vi "Excel Secondary Header Prep.vi"(0 "RefCellsIn":refnum<k7>, 7 "[IndexPageStarts]":i32[](array[numeric]), 11 "ErrorIn":errorcluster) -> (4 "RefCellsOut":refnum<k7>, 15 "ErrorOut":errorcluster)   [LabVIEW 2013]
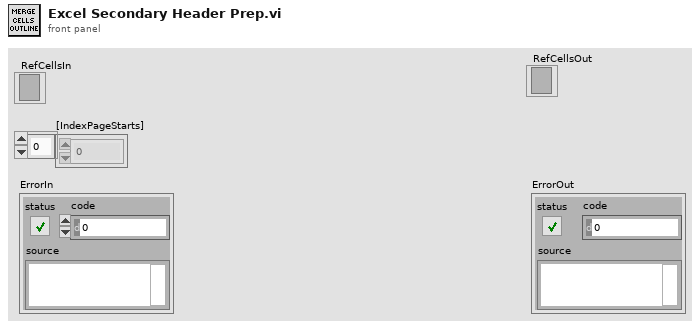
[diagram p1: front panel]
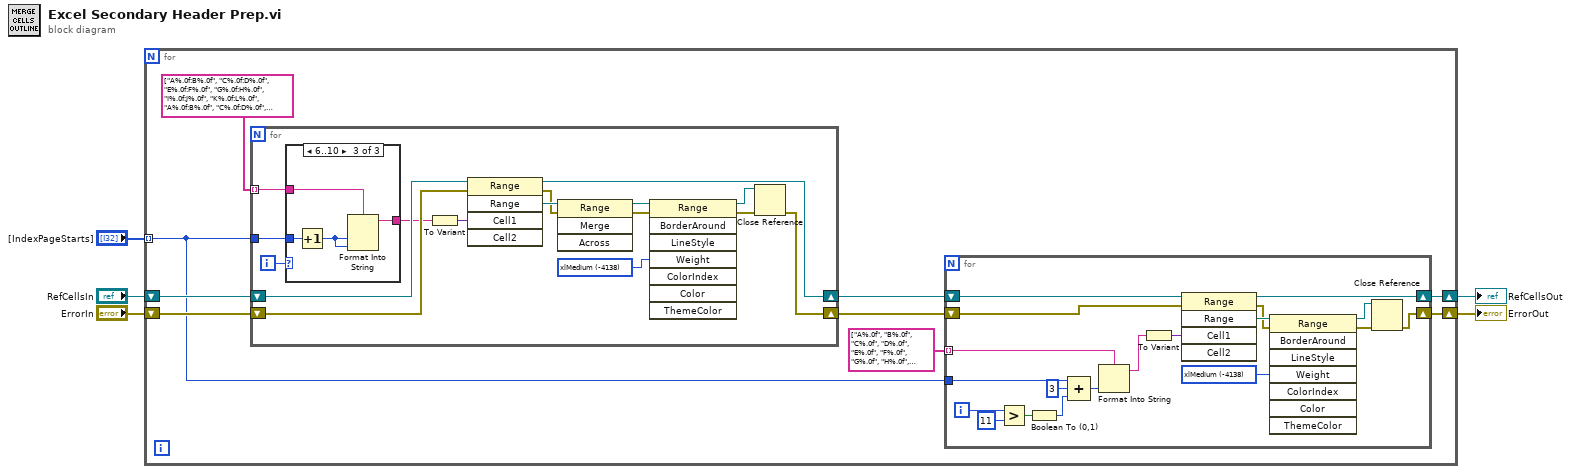
[diagram p0: block diagram]
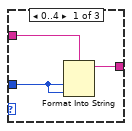
[diagram p2: hidden frame]
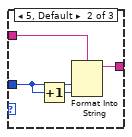
[diagram p3: hidden frame]
diagram:
  n1 = for {
    tunnel: "[IndexPageStarts]" -> [w12] mode=indexing
    shift-right: [w9] -> w3
    shift-left: "RefCellsIn" -> [w14]
    shift-right: [w8] -> w2
    shift-left: "ErrorIn" -> [w13]
    n2 = for {
      tunnel: string[] ["A%.0f:B%.0f", "C%.0f:D%.0f", "E%.0f:F%.0f", "G%.0f:H%.0f", "I%.0f:J%.0f", "K%.0f:L%.0f", "A%.0f:B%.0f", "C%.0f:D%.0f", "E%.0f:F%.0f", "G%.0f:H%.0f", "I%.0f:J%.0f"] -> [w48] mode=indexing
      tunnel: w12 -> [w47]
      shift-right: [w43] -> w11
      shift-left: w14 -> [w44]
      shift-right: [w42] -> w10
      shift-left: w13 -> [w41]
      i -> [w49]
      w39 = -4138 items=["xlHairline"=1, "xlMedium"=-4138, "xlThick"=4, "xlThin"=2] ("Weight")
      n3 = case shown="6..10" w49 {
        tunnel: w48 -> [w52 w56 w58]
        tunnel: w47 -> [w51 w55 w60]
        tunnel: [w50 w53 w57] -> w40
        frame 0..4 {
          n4 = Format Into String(format string=w52, w51, w51) -> (resulting string=w50:string)  [unwired: 2 in, 1 out]
        }
        frame 5, Default {
          n5 = Increment(x=w55) -> (x+1=w54:i32)
          n6 = Format Into String(format string=w56, w55, w54) -> (resulting string=w53:string)  [unwired: 2 in, 1 out]
        }
        frame 6..10 {
          n7 = Increment(x=w60) -> (x+1=w59:i32)
          n8 = Format Into String(format string=w58, w59, w59) -> (resulting string=w57:string)  [unwired: 2 in, 1 out]
        }
      }
      n9 = To Variant(anything=w40) -> (Variant=w34:variant)
      n10 = invoke class="Range" method="Range"(reference=w44, error in=w41, "Cell1"=w34) -> (reference out=w43:refnum<k7>, error out=w45:errorcluster, "Range"=w46:refnum<k7>)  [unwired: 2 in, 2 out]
      n11 = invoke class="Range" method="Merge"(reference=w46, error in=w45) -> (reference out=w38:refnum<k7>, error out=w37:errorcluster)  [unwired: 2 in, 2 out]
      n12 = invoke class="Range" method="BorderAround"(reference=w38, error in=w37, "Weight"=w39) -> (reference out=w36:refnum<k7>, error out=w35:errorcluster)  [unwired: 5 in, 6 out]
      n13 = Close Reference(reference=w36, error in (no error)=w35) -> (error out=w42:errorcluster)
    }
    n14 = for {
      tunnel: w12 -> [w30]
      tunnel: string[] ["A%.0f", "B%.0f", "C%.0f", "D%.0f", "E%.0f", "F%.0f", "G%.0f", "H%.0f", "I%.0f", "J%.0f", "K%.0f", "L%.0f", "A%.0f", "B%.0f", "C%.0f", "D%.0f", "E%.0f", "F%.0f", "G%.0f", "H%.0f", "I%.0f", "J%.0f", "K%.0f", "L%.0f"] -> [w26] mode=indexing
      shift-right: [w20] -> w9
      shift-left: w11 -> [w23]
      shift-right: [w15] -> w8
      shift-left: w10 -> [w22]
      i -> [w33]
      w24 = -4138 items=["xlHairline"=1, "xlMedium"=-4138, "xlThick"=4, "xlThin"=2] ("Weight")
      n15 = Greater?(x=w33, y=11) -> (0:w32:bool)
      n16 = Boolean To (0,1)(Boolean=w32) -> (0, 1=w31:i16)
      n17 = Compound Arithmetic op=unknown(w30, 3 ("value"), w31) -> (w27:i32)
      n18 = Format Into String(format string=w26, w27) -> (resulting string=w21:string)  [unwired: 2 in, 1 out]
      n19 = To Variant(anything=w21) -> (Variant=w25:variant)
      n20 = invoke class="Range" method="Range"(reference=w23, error in=w22, "Cell1"=w25) -> (reference out=w20:refnum<k7>, error out=w18:errorcluster, "Range"=w19:refnum<k7>)  [unwired: 2 in, 2 out]
      n21 = invoke class="Range" method="BorderAround"(reference=w19, error in=w18, "Weight"=w24) -> (reference out=w16:refnum<k7>, error out=w17:errorcluster)  [unwired: 5 in, 6 out]
      n22 = Close Reference(reference=w16, error in (no error)=w17) -> (error out=w15:errorcluster)
    }
  }
  "RefCellsOut" <- w3
  "ErrorOut" <- w2
